vi "Current Item.vi"(8 "error in (no error)":errorcluster caption="错误输入（无错误）", 11 "Enumerator 输入":refnum<class "Enumerator.lvclass"> caption="DNL_LabVIEW Object in") -> (0 "error out":errorcluster caption="错误输出", 2 "Item":variant, 3 "Enumerator 输出":refnum<class "Enumerator.lvclass"> caption="DNL_LabVIEW Object out")   [LabVIEW 2012, in "Enumerator.lvclass"]
uses:
  Enumerator.lvclass
  Enumerator.lvclass/Enumerator.ctl
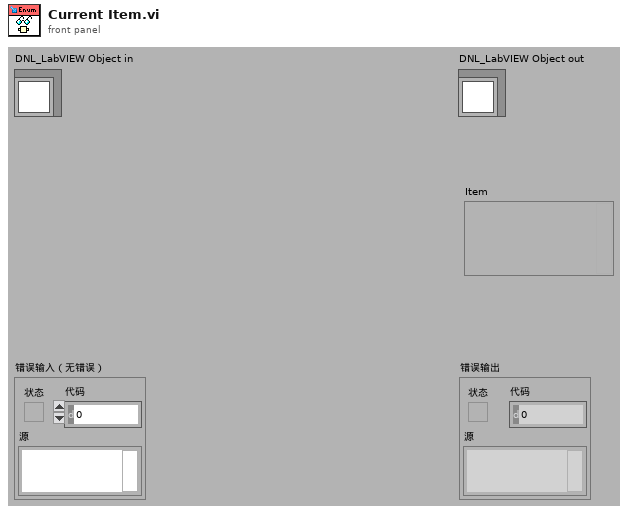
[diagram p1: front panel]
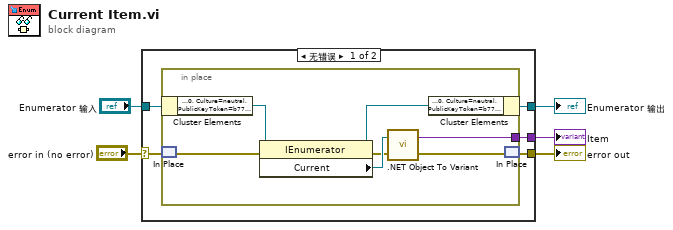
[diagram p0: block diagram]
diagram:
  n1 = case shown="无错误" "error in (no error)" {
    selector: "error in (no error)" -> [w9 w19]
    tunnel: [w8 w19] -> w4
    tunnel: [w6 w18] -> w2
    tunnel: "Enumerator 输入" -> [w10 w18]
    tunnel: [w7 _] -> w1
    frame No Error {
      n2 = in-place {
        in-place-border: [w11] -> w7
        n3 = in-place-cluster #1(w10) -> ("Enumerator"=w17:refnum<k24>)
        n4 = in-place-match #2(w9) -> (w15:errorcluster)
        n5 = property class="IEnumerator"(reference=w17, error in=w15) -> (reference out=w16:refnum<k24>, error out=w13:errorcluster, "Current"=w14:refnum<k24>)
        n6 = call <vilib>:".NET Object To Variant.vi"("error in (no error)"=w13, ".NET object"=w14) -> ("error out"=w12:errorcluster, "variant"=w11:variant)
        n7 = in-place-cluster #1("Enumerator"=w16) -> (w6:refnum<class "Enumerator.lvclass">)
        n8 = in-place-match #2(w12) -> (w8:errorcluster)
      }
    }
    frame Error {
    }
  }
  "error out" <- w4
  "Enumerator 输出" <- w2
  "Item" <- w1
